vi "Actor Core.vi"(8 "error in":errorcluster, 11 "Nested in":refnum<class "Counter ACQ.lvclass">) -> (0 "error out":errorcluster, 3 "Actor out":refnum<class "Actor.lvclass">)   [LabVIEW 2019, in "Counter ACQ.lvlib" / "Counter ACQ.lvclass"]
doc: "(<B>Filename</B>: Actor Framework.lvlib:Actor.lvclass:Actor Core.vi)\n\nReceives messages to the actor, reacts to them, and initiates any error handling that may shut the actor down.\n\nDescendant classes may override this VI to append parallel tasks for the actor to complete while it handles messages. Overrides use the Call Parent Method node."
uses:
  Counter ACQ.lvclass
  C:/Program Files/National Instruments/LabVIEW 2019/vi.lib/ActorFramework/Actor/Actor.lvclass
  <vilib>/ActorFramework/Actor/Actor.lvclass
  <vilib>/ActorFramework/Actor/Actor.lvclass/Actor.ctl
  Counter ACQ.lvclass/Counter ACQ.ctl
  Counter Messages/Leds Msg/Leds Msg.lvclass/Leds Msg.ctl
  <vilib>/ActorFramework/Message Enqueuer/Message Enqueuer.lvclass/Message Enqueuer.ctl
  <vilib>/ActorFramework/Message Enqueuer/Enqueue.vi
  <vilib>/Utility/error.llb/Clear Errors.vi
  Counter Messages/Leds Msg/Leds Msg.lvclass
  C:/Program Files/National Instruments/LabVIEW 2019/vi.lib/ActorFramework/Message/Message.lvclass
  <vilib>/ActorFramework/Stop Msg/Stop Msg.lvclass
  <vilib>/ActorFramework/Message Priority Queue/Priority Enqueue.vi
panel:
  out "x = y?":bool
  out "cuenta":dbl
  out "Start/Stop":bool
  out "Minimo":dbl
  out "Maximo":dbl
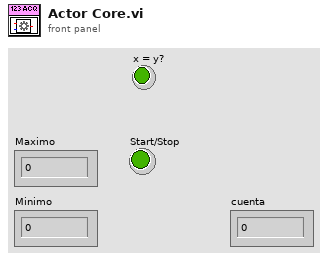
[diagram p1: front panel]
types:
  T1 = cluster{"Stop":refnum<user-event>, "Start/Stop":refnum<user-event>, "maximo":refnum<user-event>, "minimo":refnum<user-event>}
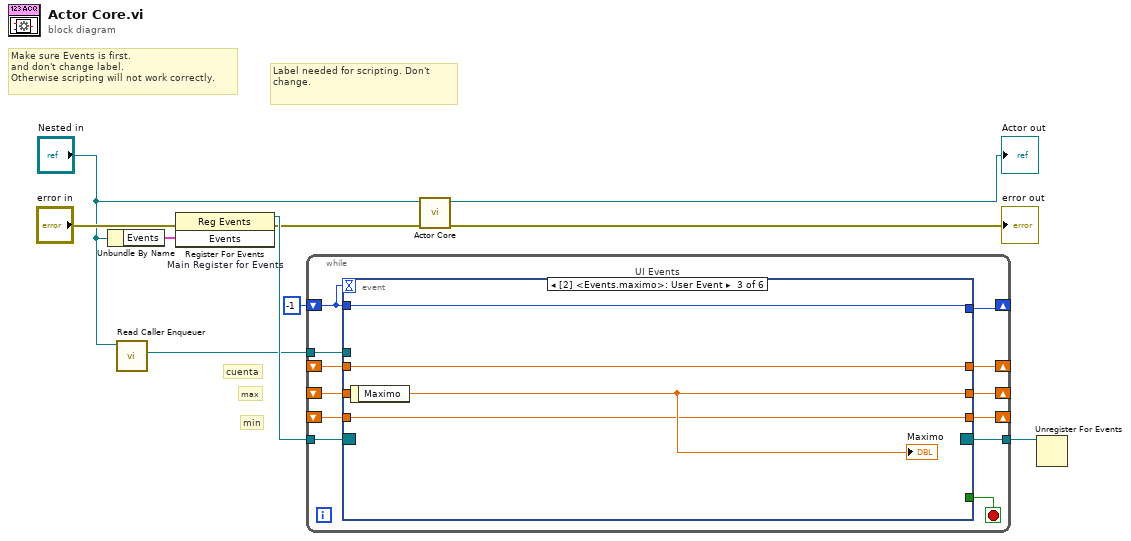
[diagram p0: block diagram]
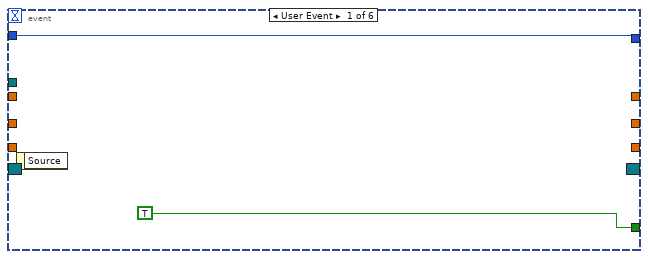
[diagram p2: hidden frame]
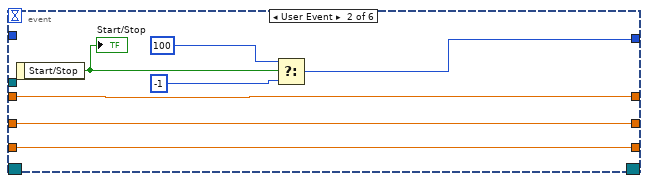
[diagram p3: hidden frame]
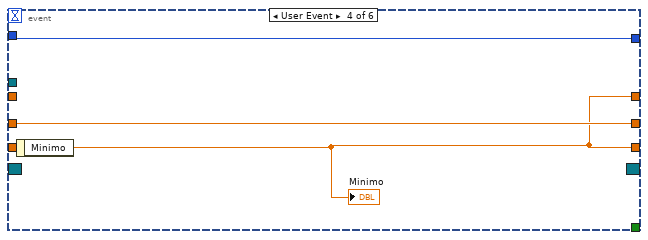
[diagram p4: hidden frame]
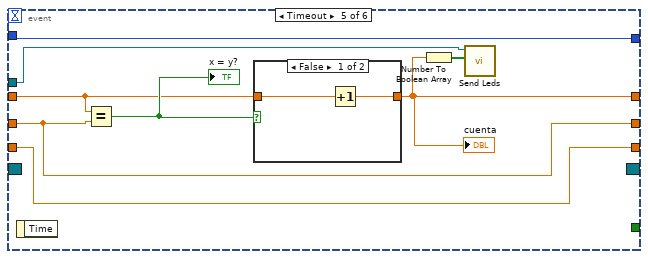
[diagram p5: hidden frame]
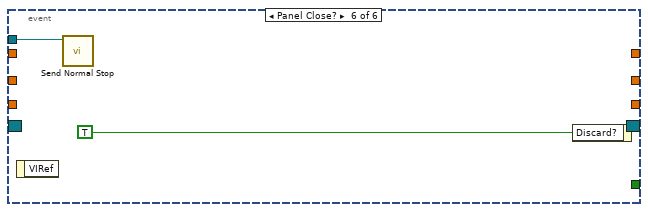
[diagram p7: hidden frame]
diagram:
  # "cuenta"
  # "min"
  # "max"
  # "Label needed for scripting. Don't change."
  # "Make sure Events is first.\nand don't change label.\nOtherwise scripting will not work correctly."
  n1 = Unbundle By Name("Nested in") -> ("Events"=w7:T1)
  n2 = call <vilib>:"Read Caller Enqueuer.vi"("Actor"="Nested in") -> ("Caller Enqueuer"=w5:refnum<class "Message Enqueuer.lvclass">)  [unwired: 10 in]
  n3 = register-events "Main Register for Events"(error in="error in", w7) -> (reference out=w8:refnum<event-registration>, error out=w3:errorcluster)  [unwired: 1 in]
  n4 = while {
    tunnel: w8 -> [w22]
    tunnel: [w20] -> w6
    tunnel: w5 -> [w19]
    shift-right: [w18] -> _
    shift-left: -1 -> [w17]
    shift-right: [w16] -> _
    shift-left: _ -> [w14]
    shift-right: [w15] -> _
    shift-left: _ -> [w13]
    shift-right: [w12] -> _
    shift-left: _ -> [w11]
    stop <- w21 stop-if-true
    n5 = event "UI Events" shown="[2] <Events.maximo>: User Event" {
      selector: w22 -> [_ _ _ _ _ _]
      dyn-events: [_ _ _ _ _ _] -> w20
      timeout: w17 -> [_ _ _ _ _ _]
      tunnel: [TRUE _ _ _ _ _] -> w21
      tunnel: w19 -> [_ _ _ _ w46 w50]
      tunnel: [w23 w29 w32 w36 w44 _] -> w18
      tunnel: w17 -> [w23 _ w32 w36 w44 _]
      tunnel: [_ w27 w35 w38 w41 _] -> w16
      tunnel: [_ w26 w34 w37 w40 _] -> w15
      tunnel: w14 -> [_ w27 _ w38 w41 _]
      tunnel: w13 -> [_ w26 w34 _ w40 _]
      tunnel: [_ w25 w33 w37 w39 _] -> w12
      tunnel: w11 -> [_ w25 w33 _ w42 _]
      event User Event {
        n6 = event-data() -> ()  [unwired: 1 in, 1 out]
      }
      event User Event {
        n7 = event-data() -> ("Start/Stop"=w28:bool)  [unwired: 1 in]
        "Start/Stop" <- w28
        n8 = Select(t=100, s=w28, f=-1) -> (s? t:f=w29:i32)
      }
      event User Event {
        n9 = event-data() -> ("Maximo"=w35:dbl)  [unwired: 1 in]
        "Maximo" <- w35
      }
      event User Event {
        n10 = event-data() -> ("Minimo"=w37:dbl)  [unwired: 1 in]
        "Minimo" <- w37
      }
      event Timeout {
        n11 = event-data() -> ()  [unwired: 1 in, 1 out]
        n12 = Equal?(x=w42, y=w41) -> (x = y?=w45:bool)
        "x = y?" <- w45
        n13 = case shown="False" w45 {
          tunnel: [w48 w49] -> w39
          tunnel: w42 -> [w47 w49]
          frame False {
            n14 = Increment(x=w47) -> (x+1=w48:dbl)
          }
          frame True {
          }
        }
        "cuenta" <- w39
        n15 = Number To Boolean Array(number=w39) -> (Boolean array=w43:bool[])
        n16 = call "Send Leds.vi"("leds"=w43, "Message Enqueuer"=w46) -> ()  [unwired: 8 in, 2 out]
      }
      event Panel Close? {
        n17 = event-data() -> ()  [unwired: 1 in, 1 out]
        n18 = call <vilib>:"Send Normal Stop.vi"("Message Enqueuer"=w50) -> ()  [unwired: 10 in, 1 out]
        n19 = event-data("Discard?"=TRUE) -> ()  [unwired: 1 in, 1 out]
      }
    }
  }
  n20 = call-parent "Actor Core.vi"("error in"=w3, "Actor in"="Nested in") -> ("error out"=→"error out":errorcluster, "Actor out"=→"Actor out":refnum<class "Actor.lvclass">)  [unwired: 8 in]
  n21 = Unregister For Events(event registration refnum=w6) -> ()  [unwired: 1 in, 1 out]
